vi "Load DBC.vi"(8 "error in":errorcluster, 9 "Cluster Name":string, 10 "DBC File":string, 11 "DBCCommunication in":refnum<class "DBC Communicator.lvclass">) -> (0 "error out":errorcluster, 3 "DBCCommunication out":refnum<class "DBC Communicator.lvclass">)   [LabVIEW 2024, in "DBC Communicator.lvclass"]
uses:
  DBC Communicator.lvclass
  <resource>/objmgr/xnet.rc
  <vilib>/xnet/xnet.llb/XNET Create Session (Conversion).vi
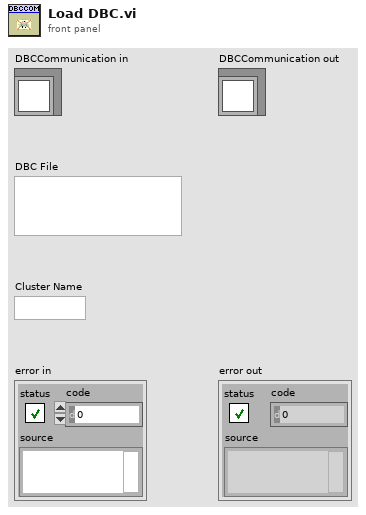
[diagram p1: front panel]
types:
  T1 = typedef "DBC Communicator.lvclass/ObjectAttributes.ctl" = cluster{"XNET Conversion Session":refnum<k21>, "Frame ID - Timestamp":map{u32, timestamp}, "Signals":cluster{"Names":string[], "Frame IDs":u32[]}}
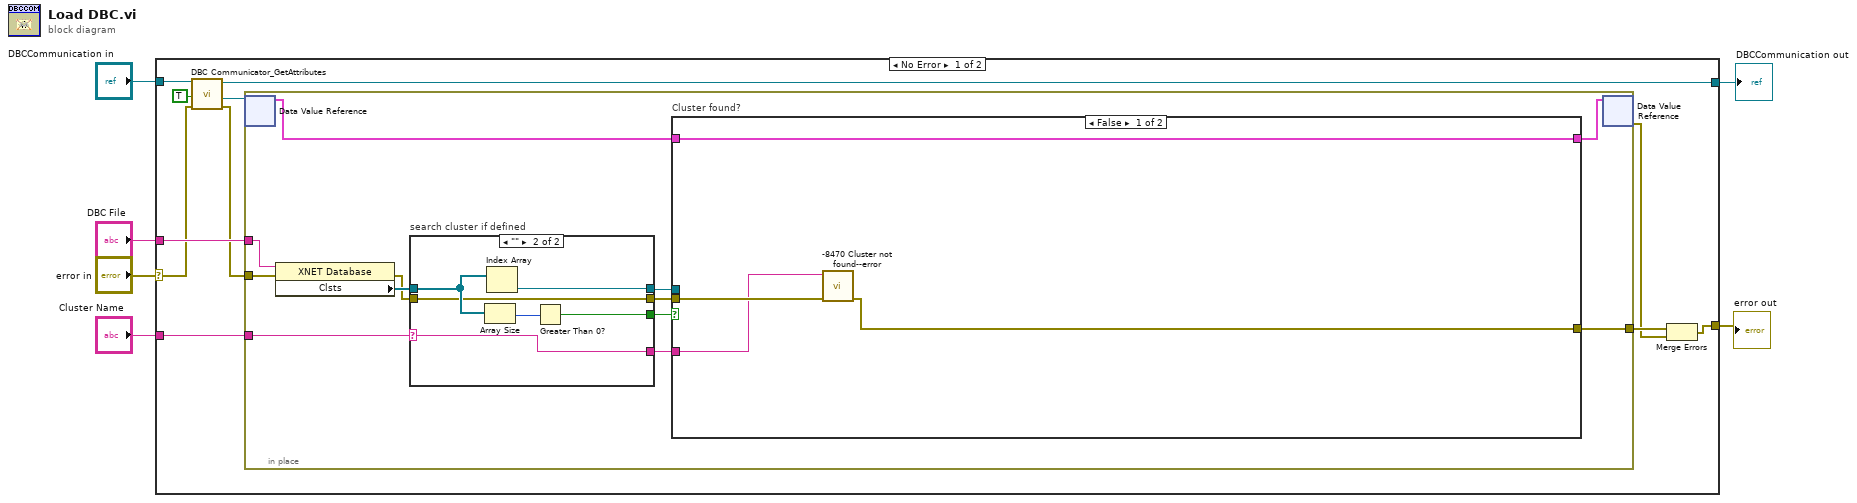
[diagram p0: block diagram]
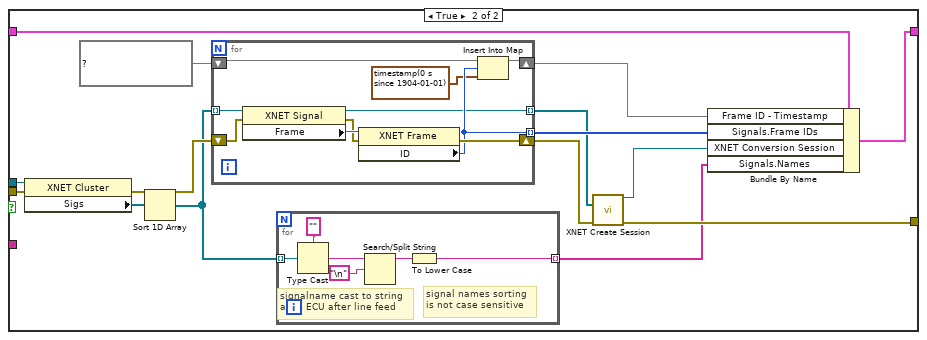
[diagram p2: hidden frame]
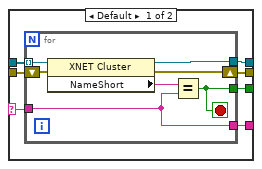
[diagram p3: hidden frame]
diagram:
  n1 = case shown="No Error" "error in" {
    selector: "error in" -> [w11 w85]
    tunnel: "DBC File" -> [w17 _]
    tunnel: "Cluster Name" -> [w15 _]
    tunnel: "DBCCommunication in" -> [w14 w86]
    tunnel: [w9 w86] -> w2
    tunnel: [w8 w85] -> w1
    frame No Error {
      n2 = call "DBC Communicator_GetAttributes.vi"("Error In"=w11, "OnlyGetDvrReference(False)"=TRUE, "reference in"=w14) -> ("Error Out"=w10:errorcluster, "DataRef"=w13:refnum<data-value>, "reference out"=w9:refnum<class "DBC Communicator.lvclass">)  [unwired: 5 in, 1 out]
      n3 = in-place {
        in-place-border: w10 -> [w29]
        in-place-border: w17 -> [w20]
        in-place-border: [w28] -> w16
        in-place-border: w15 -> [w23]
        n4 = in-place-dvr #1(w13) -> (w19:T1)  [unwired: 1 out]
        n5 = property class="XNET Database"(reference=w20, error in=w29) -> (error out=w26:errorcluster, "Clsts"=w27:refnum<k21>[])  [unwired: 1 out]
        n6 = case "search cluster if defined" shown="\"\"" w23 {
          selector: w23 -> [w70 w80]
          tunnel: w27 -> [w71 w83]
          tunnel: [w69 w84] -> w24
          tunnel: [w68 w81] -> w22
          tunnel: [w67 w80] -> w21
          tunnel: w26 -> [w66 w79]
          tunnel: [w65 w79] -> w25
          frame Default {
            n7 = for {
              tunnel: [w78] -> w69
              tunnel: w71 -> [w77] mode=indexing
              tunnel: w70 -> [w74]
              tunnel: [w75] -> w68
              tunnel: [w74] -> w67
              shift-right: [w72] -> w65
              shift-left: w66 -> [w73]
              stop <- w75 stop-if-true
              n8 = property class="XNET Cluster"(reference=w77, error in=w73) -> (reference out=w78:refnum<k21>, error out=w72:errorcluster, "NameShort"=w76:string)
              n9 = Equal?(x=w76, y=w74) -> (x = y?=w75:bool)
            }
          }
          frame "" {
            n10 = Array Size(array=w83) -> (size(s)=w82:i32)
            n11 = Index Array(array=w83) -> (element=w84:refnum<k21>)  [unwired: 1 in]
            n12 = Greater Than 0?(x=w82) -> (x > 0?=w81:bool)
          }
        }
        n13 = case "Cluster found?" shown="False" w22 {
          tunnel: w19 -> [w33 w47]
          tunnel: [w33 w45] -> w18
          tunnel: [w31 w37] -> w28
          tunnel: w25 -> [w32 w44]
          tunnel: w24 -> [_ w43]
          tunnel: w21 -> [w30 _]
          frame False {
            n14 = call "-8470 Cluster not found--error.vi"("error in"=w32, "Cluster Name"=w30) -> ("error out"=w31:errorcluster)  [unwired: 9 in]
          }
          frame True {
            n15 = property class="XNET Cluster"(reference=w43, error in=w44) -> (error out=w42:errorcluster, "Sigs"=w48:refnum<k21>[])  [unwired: 1 out]
            n16 = Sort 1D Array(array=w48) -> (sorted array=w36:refnum<k21>[])
            n17 = for {
              tunnel: w36 -> [w64] mode=indexing
              shift-right: [w60] -> w38
              shift-left: w42 -> [w61]
              tunnel: [w58] -> w41 mode=indexing
              shift-right: [w56] -> w40
              shift-left: map{u32, timestamp} {} ("Size: 0") -> [w59]
              tunnel: [w55] -> w34 mode=indexing
              n18 = property class="XNET Signal"(reference=w64, error in=w61) -> (reference out=w55:refnum<k21>, error out=w62:errorcluster, "Frame"=w63:refnum<k21>)
              n19 = property class="XNET Frame"(reference=w63, error in=w62) -> (error out=w60:errorcluster, "ID"=w58:u32)  [unwired: 1 out]
              n20 = Insert Into Map(map in=w59, key=w58, value=timestamp(0 s since 1904-01-01)) -> (map out=w56:map{u32, timestamp})  [unwired: 2 out]
            }
            n21 = for {
              tunnel: w36 -> [w53] mode=indexing
              tunnel: [w49] -> w35 mode=indexing
              # "signal names sorting\nis not case sensitive"
              # "signalname cast to string\nadds ECU after line feed"
              n22 = Type Cast(type="", x=w53) -> (*(type *) &x=w52:string)
              n23 = Search/Split String(string=w52, search string/char (-)="\n") -> (substring before match=w50:string)  [unwired: 1 in, 2 out]
              n24 = To Lower Case(string=w50) -> (all lower case string=w49:string)
            }
            n25 = call-poly <vilib>:"XNET Create Session.vi"("signal list"=w34, "error in (no error)"=w38) -> ("session out"=w46:refnum<k21>, "error out"=w37:errorcluster)  [unwired: 12 in]
            n26 = Bundle By Name(cluster=w47, "Frame ID - Timestamp"=w40, "Signals.Frame IDs"=w41, "XNET Conversion Session"=w46, "Signals.Names"=w35) -> (w45:T1)
          }
        }
        n27 = in-place-dvr #1(w18) -> (w7:errorcluster)  [unwired: 1 out]
      }
      n28 = Merge Errors(w16, w7) -> (w8:errorcluster)
    }
    frame Error {
    }
  }
  "error out" <- w1
  "DBCCommunication out" <- w2
